vi "System UI.vi"() -> ()   [LabVIEW 2025, in "System.lvlib" / "System.lvclass"]
doc: "Copyright 2017 National Instruments Corporation\n\nLicensed under the Apache License, Version 2.0 (the \"License\"); you may not use this file except in compliance with the License. You may obtain a copy of the License at http://www.apache.org/licenses/LICENSE-2.0\nUnless required by applicable law or agreed to in writing, software distributed under the License is distributed on an \"AS IS\" BASIS, WITHOUT WARRANTIES OR CONDITIONS OF ANY KIND, either express or implied. See the License for the specific language governing permissions and limitations under the License."
uses:
  System.lvclass
  Users/Public/Documents/Sandia National Labs/TSS Plugin/CEF.lvlibp/Node/mainQref.ctl
  Users/Public/Documents/Sandia National Labs/TSS Plugin/CEF.lvlibp/Node/UserEventRef.ctl
  System configuration/System.ctl
  Users/Public/Documents/Sandia National Labs/TSS Plugin/CEF.lvlibp/Node/NodeRef.ctl
  Users/Public/Documents/Sandia National Labs/TSS Plugin/CEF.lvlibp/Node/CEF_Node.lvclass
  System.lvclass/System.ctl
  System configuration/System configuration.lvclass/System configuration.ctl
  System configuration/Read System.vi
  System configuration/Write System.vi
  System configuration/System configuration.lvclass
panel:
  in  "node ref":T1
  in  "System":T2={"System Info"={"Project"="", "Program"="W87-1", "Test Name"="No name", "Serial Number"="001", "Plugin"=path "C:/Users/Public/Documents/Sandia National Labs/TSS Plugin", "Glyphs"=path "C:/Users/Public/Documents/Sandia National Labs/Glyphs"}, "Part Info"=0}
  in  "user event":T3
  in  "main queue":T4
  # "Use shorthand name at Test Info"
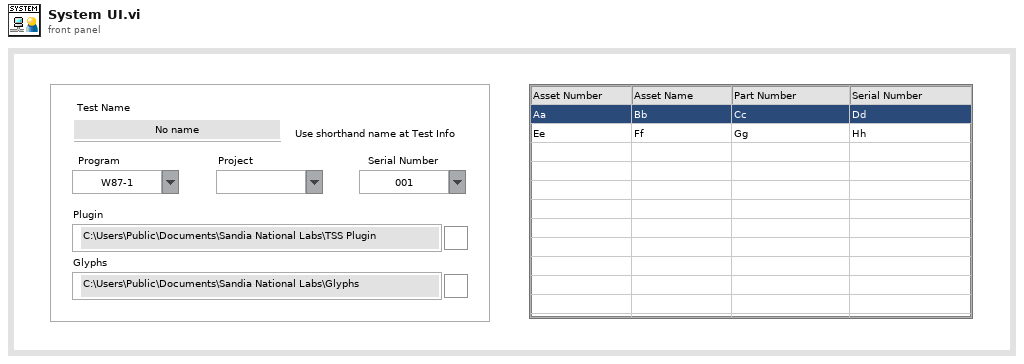
[diagram p1: front panel]
types:
  T1 = typedef "CEF.lvlibp/CEF_Node.lvclass/NodeRef.ctl" = refnum<data-value>
  T2 = typedef "System.lvlib/System configuration.lvclass/System.ctl" = cluster{"System Info":cluster{"Project":string, "Program":string, "Test Name":string, "Serial Number":string, "Plugin":path, "Glyphs":path}, "Part Info":i32}
  T3 = typedef "CEF.lvlibp/CEF_Node.lvclass/UserEventRef.ctl" = refnum<user-event>
  T4 = typedef "CEF.lvlibp/CEF_Node.lvclass/mainQref.ctl" = refnum<queue>
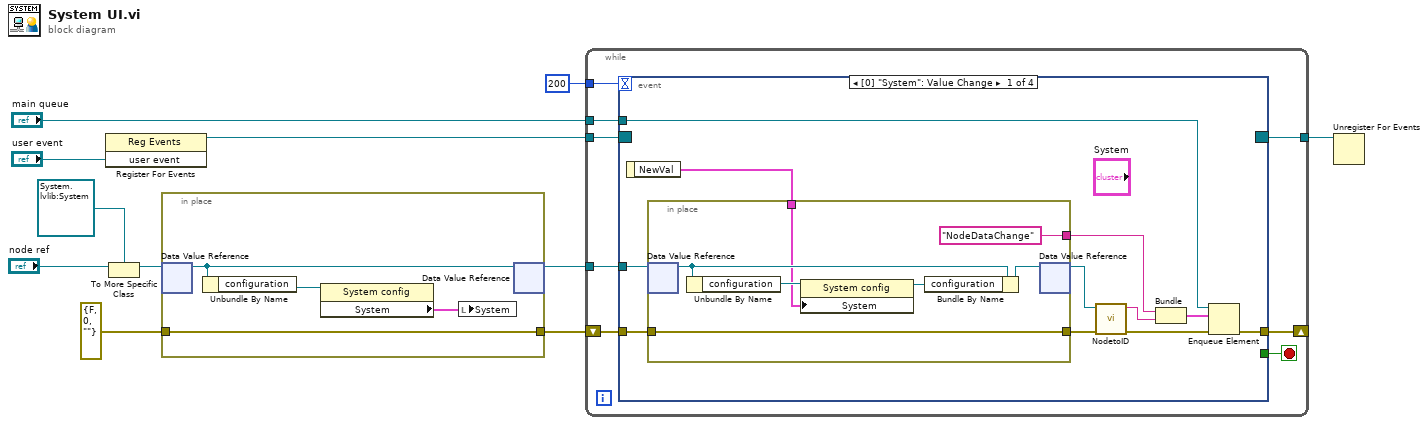
[diagram p0: block diagram]
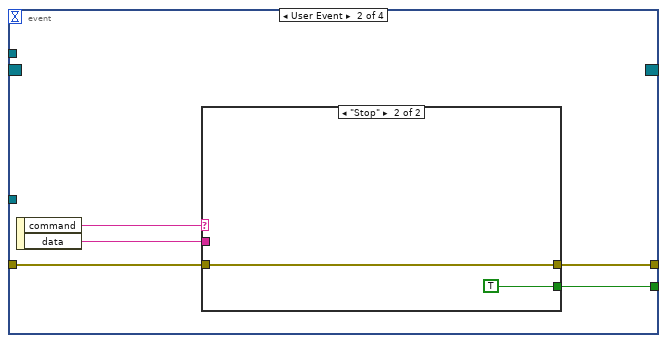
[diagram p2: hidden frame]
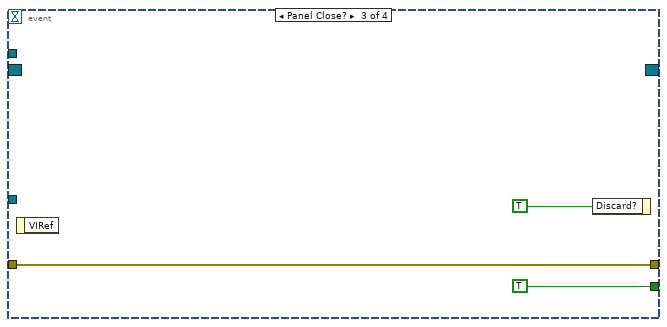
[diagram p4: hidden frame]
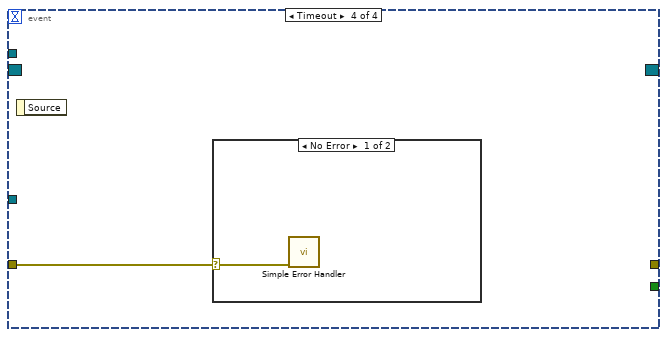
[diagram p5: hidden frame]
diagram:
  n1 = register-events("user event") -> (reference out=w6:refnum<event-registration>)  [unwired: 2 in, 1 out]
  n2 = To More Specific Class(target class=refnum<data-value> refnum ("data value reference"), reference="node ref") -> (specific class reference=w8:refnum<data-value>)  [unwired: 1 in, 1 out]
  n3 = in-place {
    in-place-border: errorcluster {"status"=FALSE, "code"=0, "source"=""} ("error out") -> [w12]
    in-place-border: [w12] -> w3
    n4 = in-place-dvr #1(w8) -> (w15:refnum<class "System.lvclass">)  [unwired: 1 out]
    n5 = Unbundle By Name(w15) -> ("configuration"=w14:refnum<class "System configuration.lvclass">)
    n6 = property class="System config"(reference=w14) -> ("System"=w13:T2)  [unwired: 1 in, 2 out]
    n7 = local write "System"(w13) -> ()
    n8 = in-place-dvr #1(w15) -> (w11:refnum<data-value>)  [unwired: 1 out]
  }
  n9 = while {
    tunnel: w6 -> [w21]
    tunnel: "main queue" -> [w18]
    tunnel: w11 -> [w20]
    tunnel: 200 -> [w17]
    shift-right: [w22] -> _
    shift-left: w3 -> [w23]
    tunnel: [w16] -> w5
    stop <- w19 stop-if-true
    n10 = event shown="[0] \"System\": Value Change" {
      selector: w21 -> [_ _ _ _]
      dyn-events: [_ _ _ _] -> w16
      timeout: w17 -> [_ _ _ _]
      tunnel: w23 -> [w29 w44 w52 w53]
      tunnel: [w32 w43 w52 _] -> w22
      tunnel: w20 -> [w34 _ _ _]
      tunnel: [_ w45 TRUE _] -> w19
      tunnel: w18 -> [w31 _ _ _]
      event Value Change {
        n11 = event-data() -> ("NewVal"=w27:T2)  [unwired: 1 out]
        n12 = in-place {
          in-place-border: w29 -> [w35]
          in-place-border: [w35] -> w28
          in-place-border: w27 -> [w36]
          in-place-border: ["NodeDataChange" ("Message Name")] -> w26
          n13 = in-place-dvr #2(w34) -> (w41:refnum<class "System.lvclass">)  [unwired: 1 out]
          n14 = Unbundle By Name(w41) -> ("configuration"=w37:refnum<class "System configuration.lvclass">)
          n15 = property class="System config"(reference=w37, "System"=w36) -> (reference out=w39:refnum<class "System configuration.lvclass">)  [unwired: 1 in, 1 out]
          n16 = Bundle By Name(cluster=w41, "configuration"=w39) -> (w40:refnum<class "System.lvclass">)
          n17 = in-place-dvr #2(w40) -> (w30:refnum<data-value>)  [unwired: 1 out]
        }
        n18 = call "NodetoID.vi"("error in"=w28, "node ref"=w30) -> ("error out"=w33:errorcluster, "ID"=w25:string)  [unwired: 8 in]
        n19 = Bundle("Message Name"=w26, "ID"=w25) -> (w24:cluster{"Message Name":string, "ID":string})  [unwired: 1 in]
        n20 = Enqueue Element(queue=w31, element=w24, error in (no error)=w33) -> (error out=w32:errorcluster)  [unwired: 1 in, 2 out]
      }
      event User Event {
        n21 = event-data() -> ("command"=w46:string, "data"=w42:string)  [unwired: 1 out]
        n22 = case shown="\"Stop\"" w46 {
          tunnel: [_ TRUE] -> w45
          tunnel: w44 -> [w47 w48]
          tunnel: [w47 w48] -> w43
          tunnel: w42 -> [_ _]
          frame Default {
          }
          frame "Stop" {
          }
        }
      }
      event Panel Close? {
        n23 = event-data() -> ()  [unwired: 2 out]
        n24 = event-data("Discard?"=TRUE) -> ()  [unwired: 1 in, 1 out]
      }
      event Timeout {
        n25 = event-data() -> ()  [unwired: 2 out]
        n26 = case shown="No Error" w53 {
          selector: w53 -> [w54 _]
          frame No Error {
            n27 = call <vilib>:"Simple Error Handler.vi"("error in (no error)"=w54) -> ()  [unwired: 4 in, 5 out]
          }
          frame Error {
          }
        }
      }
    }
  }
  n28 = Unregister For Events(event registration refnum=w5) -> ()  [unwired: 1 in, 1 out]
